vi "CCM-Register Events.vi"(7 "Conn Refs":refnum<vi>[](array[refnum]), 9 "DE List":refnum<vi>, 10 "List Refs":refnum<vi>[](array[refnum]), 11 "Table Refs":refnum<vi>[](array[refnum])) -> (1 "Lists":T4, 2 "Tables":cluster{"DO":T2, "DI":T2}, 3 "Event Registration Refnum":refnum<event-registration>)   [LabVIEW 2020]
uses:
  Utility VIs/Controls/KListboxEx/KListboxEx.xctl
  Utility VIs/Controls/KTable/KTable.xctl
  Utility VIs/Controls/KListboxEx/Events.ctl
  Utility VIs/Controls/KListboxEx/Event Action.ctl
  Utility VIs/Controls/KTable/Events.ctl
  Utility VIs/Controls/KTable/Event Data.ctl
  Utility VIs/Controls/KTable/Event Type.ctl
  Type Defs/General PXISlot XControl/PXISlotGP.xctl
  Type Defs/PXISlot XControl/Connector Type.ctl
panel:
  out "Slot":T1
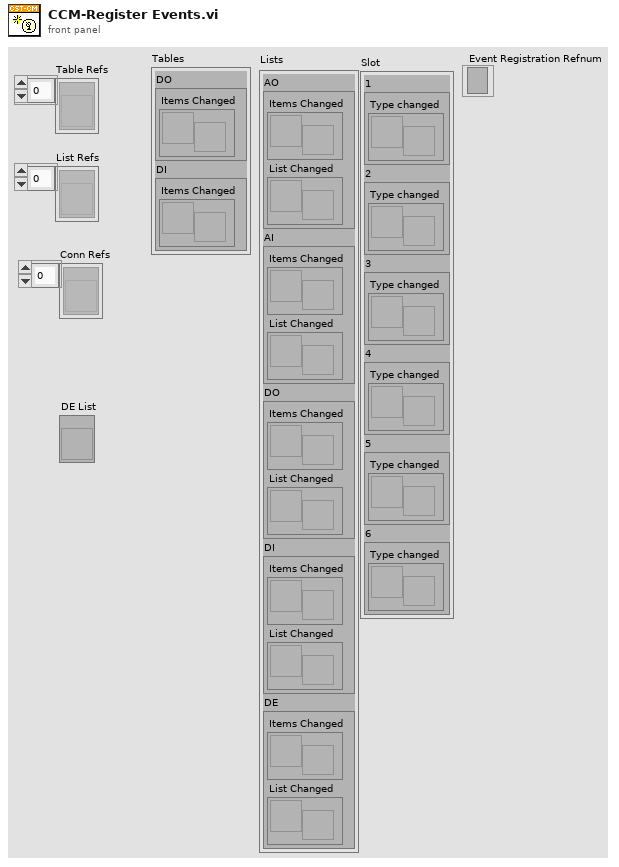
[diagram p1: front panel]
types:
  T1 = cluster{"1":cluster{"Type changed":refnum<user-event>}, "2":cluster{"Type changed":refnum<user-event>}, "3":cluster{"Type changed":refnum<user-event>}, "4":cluster{"Type changed":refnum<user-event>}, "5":cluster{"Type changed":refnum<user-event>}, "6":cluster{"Type changed":refnum<user-event>}}
  T2 = typedef "KTable.xctl/Events.ctl" = cluster{"Items Changed":refnum<user-event>}
  T3 = typedef "KListboxEx.xctl/Events.ctl" = cluster{"Items Changed":refnum<user-event>, "List Changed":refnum<user-event>}
  T4 = cluster{"AO":T3, "AI":T3, "DO":T3, "DI":T3, "DE":T3}
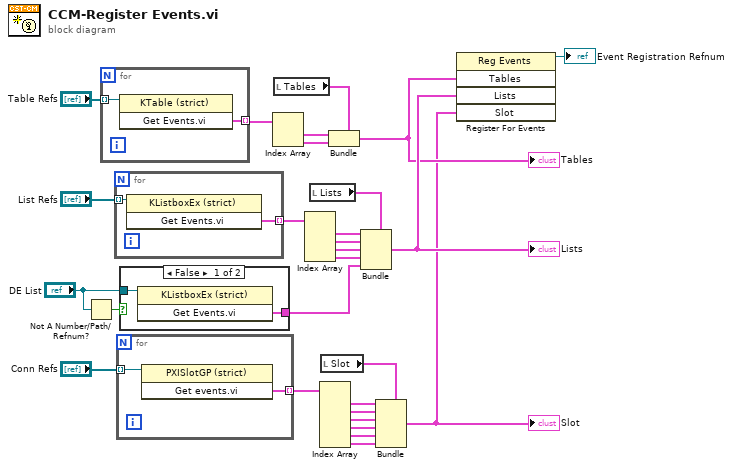
[diagram p0: block diagram]
diagram:
  n1 = Not A Number/Path/Refnum?(number/path/refnum="DE List") -> (NaN/Path/Refnum?=w1:bool)
  n2 = for {
    tunnel: "Table Refs" -> [w30] mode=indexing
    tunnel: [w29] -> w17 mode=indexing
    n3 = invoke class="KTable (strict)" method="Get Events.vi"(reference=w30) -> ("Get Events.vi"=w29:T2)  [unwired: 2 in, 2 out]
  }
  n4 = for {
    tunnel: "List Refs" -> [w32] mode=indexing
    tunnel: [w31] -> w25 mode=indexing
    n5 = invoke class="KListboxEx (strict)" method="Get Events.vi"(reference=w32) -> ("Get Events.vi"=w31:T3)  [unwired: 2 in, 2 out]
  }
  n6 = for {
    tunnel: "Conn Refs" -> [w34] mode=indexing
    tunnel: [w33] -> w7 mode=indexing
    n7 = invoke class="PXISlotGP (strict)" method="Get events.vi"(reference=w34) -> ("Get events.vi"=w33:cluster{"Type changed":refnum<user-event>})  [unwired: 2 in, 2 out]
  }
  n8 = case shown="False" w1 {
    tunnel: "DE List" -> [w36 _]
    tunnel: [w35 _] -> w4
    frame False {
      n9 = invoke class="KListboxEx (strict)" method="Get Events.vi"(reference=w36) -> ("Get Events.vi"=w35:T3)  [unwired: 2 in, 2 out]
    }
    frame True {
    }
  }
  n10 = Index Array(array=w17) -> (element #1=w19:T2, element #2=w18:T2)  [unwired: 2 in]
  n11 = local read "Tables"() -> (w16:cluster{"DO":T2, "DI":T2})
  n12 = Index Array(array=w25) -> (element #1=w24:T3, element #2=w23:T3, element #3=w22:T3, element #4=w21:T3)  [unwired: 4 in]
  n13 = local read "Lists"() -> (w26:T4)
  n14 = Index Array(array=w7) -> (element #1=w13:cluster{"Type changed":refnum<user-event>}, element #2=w12:cluster{"Type changed":refnum<user-event>}, element #3=w11:cluster{"Type changed":refnum<user-event>}, element #4=w10:cluster{"Type changed":refnum<user-event>}, element #5=w9:cluster{"Type changed":refnum<user-event>}, element #6=w8:cluster{"Type changed":refnum<user-event>})  [unwired: 6 in]
  n15 = local read "Slot"() -> (w6:T1)
  n16 = Bundle(cluster=w16, "DO"=w19, "DI"=w18) -> (w15:cluster{"DO":T2, "DI":T2})
  "Tables" <- w15
  n17 = Bundle(cluster=w26, "AO"=w24, "AI"=w23, "DO"=w22, "DI"=w21, "DE"=w4) -> (w20:T4)
  "Lists" <- w20
  n18 = Bundle(cluster=w6, "1"=w13, "2"=w12, "3"=w11, "4"=w10, "5"=w9, "6"=w8) -> (w5:T1)
  "Slot" <- w5
  n19 = register-events(w15, w20, w5) -> (reference out=→"Event Registration Refnum":refnum<event-registration>)  [unwired: 2 in, 1 out]
